vi "ET_Example.vi"() -> ()   [LabVIEW 2016]
uses:
  Source/Methods/Envelope Tracking/Typedefs/Detrough Configuration.ctl
  Source/Methods/Envelope Tracking/Typedefs/Detrough Type.ctl
  Source/SG/Typedefs/Instrument Configuration.ctl
  <instrlib>/niRFSG/niRFSG.llb/niRFSG Ref Clock Sources.ctl
  Source/Common/Local Oscillator Sharing Mode.ctl
  Source/Methods/Envelope Tracking/Typedefs/Synchronization Configuration.ctl
  Source/Methods/Envelope Tracking/Typedefs/Envelope Generator Configuration.ctl
  Source/Methods/Envelope Tracking/Typedefs/Tracker Configuration.ctl
  Source/Methods/Envelope Tracking/Typedefs/Lookup Table Configuration.ctl
  <instrlib>/niRFSG/niRFSG.llb/niRFSG Exported Signal Destinations.ctl
  Source/SG/SG.lvlib
  Source/Methods/Envelope Tracking/Envelope Tracking.lvlib
  Source/Common/Common.lvlib
panel:
  in  "stop":bool
  out "Status":string="Initializing..."
  out "error out":errorcluster {"code" format="%.0x"}
  in  "Configuration":T1(tab)
  in  "RF Signal Generator":refnum<k15>="5840"
  in  "Tracker Signal Generator":refnum<k15>="5820"
  in  "Waveform File Path":path=path "C:/Users/Public/Documents/National Instruments/RFIC Test Software/Waveforms/LTE_FDD_DL_1x20MHz_TM11_OS4.tdms"
  in  "Synchronization Configuration":T2={"RF Delay Range (s)"=1.9999999949504854e-06, "RF Delay (s)"=0.0} {"RF Delay (s)" format="%#_6p"; "RF Delay Range (s)" format="%#_6p"}
  in  "SG Configuration":T3={"SelectedPorts"="", "Reference Clock Source"="PXI_CLK", "Carrier Frequency (Hz)"=1000000000.0, "DUT Average Input Power (dBm)"=-10.0, "External Attenuation (dB)"=0.0, "LO Sharing Mode"=enum."Automatic"} {"Carrier Frequency (Hz)" format="%#_6p"}
  in  "Envelope Generator Configuration":T6={"Reference Clock Source"="PXI_CLK"}
  in  "Tracker Configuration":T7={"Input Impedance (Ohms)"=1000000.0, "Common Mode Offset (V)"=1.0, "Gain (V/V)"=2.5, "Output Offset (V)"=2.55} {"Input Impedance (Ohms)" format="%#_6p"}
  in  "Tracker Start Trigger Export":T8="PFI0"
  in  "Envelope Method":enum32{"Detrough", "LUT"}(tab)=enum."LUT"
  in  "Detrough Configuration":T9={"Type"=enum."Exponential", "Minimum Voltage (V)"=1.5, "Maximum Voltage (V)"=3.5, "Exponent"=1.2000000476837158}
  in  "Lookup Table Configuration":T11={"DUT Average Input Power (dBm)"=0.0, "DUT Input Power (dBm)"=array[1024 elements], "Supply Voltage (V)"=array[1024 elements]}
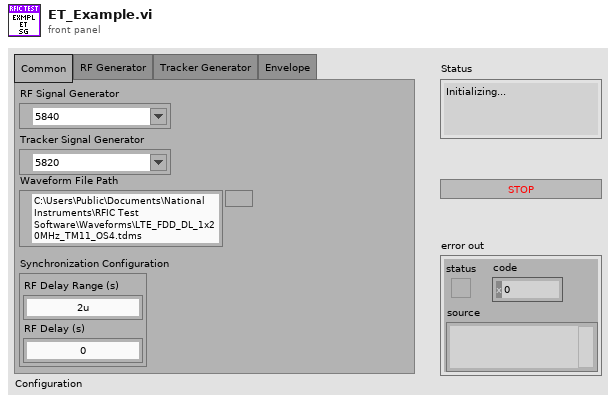
[diagram p1: front panel]
types:
  T1 = enum32{"Common", "RF Generator", "Tracker Generator", "Envelope"}
  T2 = typedef "Envelope Tracking.lvlib/Synchronization Configuration.ctl" = cluster{"RF Delay Range (s)":dbl, "RF Delay (s)":dbl}
  T3 = typedef "SG.lvlib/Instrument Configuration.ctl" = cluster{"SelectedPorts":string, "Reference Clock Source":T4, "Carrier Frequency (Hz)":dbl, "DUT Average Input Power (dBm)":dbl, "External Attenuation (dB)":dbl, "LO Sharing Mode":T5}
  T4 = typedef "niRFSG Ref Clock Sources.ctl" = string
  T5 = typedef "Common.lvlib/Local Oscillator Sharing Mode.ctl" = enum16{"Automatic", "None"}
  T6 = typedef "Envelope Tracking.lvlib/Envelope Generator Configuration.ctl" = cluster{"Reference Clock Source":T4}
  T7 = typedef "Envelope Tracking.lvlib/Tracker Configuration.ctl" = cluster{"Input Impedance (Ohms)":dbl, "Common Mode Offset (V)":dbl, "Gain (V/V)":dbl, "Output Offset (V)":dbl}
  T8 = typedef "niRFSG Exported Signal Destinations.ctl" = string
  T9 = typedef "Envelope Tracking.lvlib/Detrough Configuration.ctl" = cluster{"Type":T10, "Minimum Voltage (V)":dbl, "Maximum Voltage (V)":dbl, "Exponent":dbl}
  T10 = typedef "Envelope Tracking.lvlib/Detrough Type.ctl" = enum16{"Exponential", "Cosine", "Power"}
  T11 = typedef "Envelope Tracking.lvlib/Lookup Table Configuration.ctl" = cluster{"DUT Average Input Power (dBm)":dbl, "DUT Input Power (dBm)":sgl[], "Supply Voltage (V)":sgl[]}
  T12 = typedef "Common.lvlib/Waveform.ctl" = cluster{"Name":string, "Data":refnum<data-value>, "Signal Bandwidth (Hz)":dbl, "PAPR (dB)":dbl, "Burst Length (s)":dbl, "Sample Rate":dbl, "Burst Start Locations":i32[], "Burst Stop Locations":i32[], "Idle Duration Present?":bool, "Runtime Scaling":dbl, "Script":string}
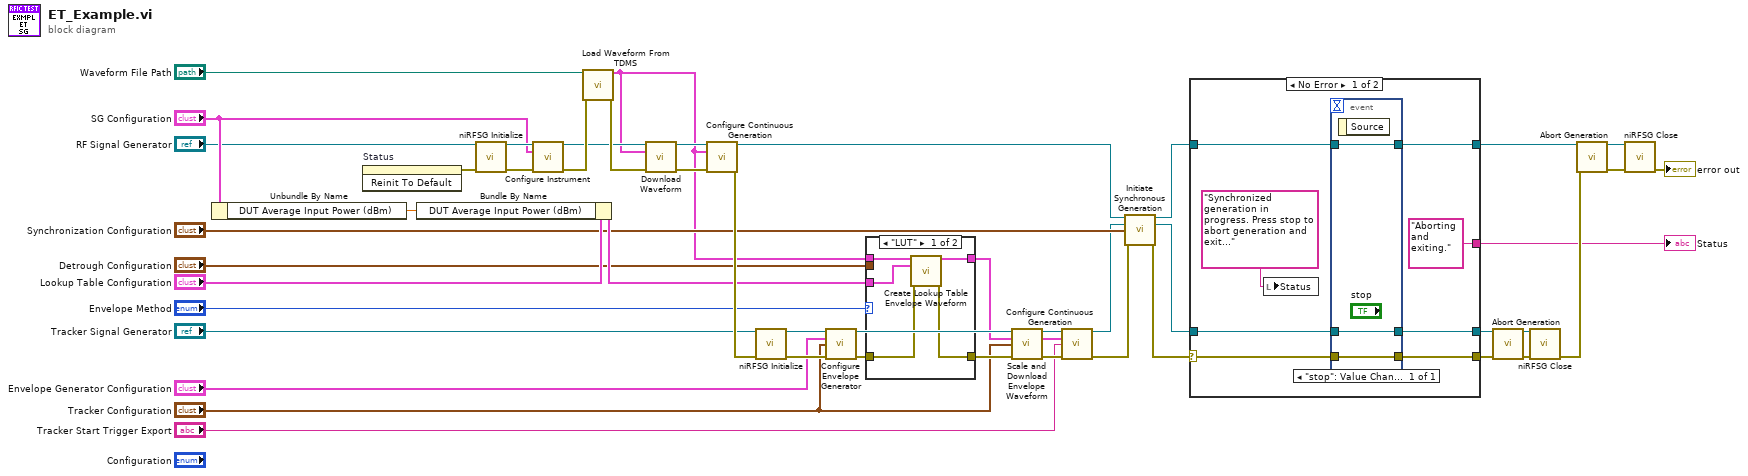
[diagram p0: block diagram]
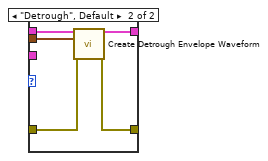
[diagram p2: hidden frame]
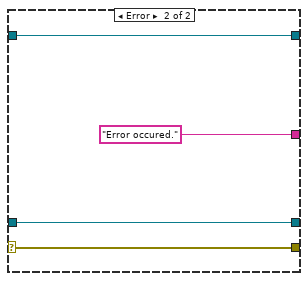
[diagram p3: hidden frame]
diagram:
  n1 = Unbundle By Name("SG Configuration") -> ("DUT Average Input Power (dBm)"=w3:dbl)
  n2 = invoke on="Status" class="Str" method="Reinit To Default"() -> (error out=w32:errorcluster)  [unwired: 3 in, 2 out]
  n3 = Bundle By Name(cluster="Lookup Table Configuration", "DUT Average Input Power (dBm)"=w3) -> (w30:T11)
  n4 = call <instrlib>:"niRFSG Initialize.vi"("resource name"="RF Signal Generator", "error in"=w32) -> ("instrument handle"=w27:refnum<k15>, "error out"=w48:errorcluster)  [unwired: 12 in]
  n5 = call "Configure Instrument.vi"("RFSG Session In"=w27, "SG Configuration"="SG Configuration", "error in (no error)"=w48) -> ("RFSG Session Out"=w26:refnum<k15>, "error out"=w40:errorcluster)  [unwired: 11 in]
  n6 = call "Load Waveform From TDMS.vi"("TDMS File Path"="Waveform File Path", "error in (no error)"=w40) -> ("Waveform"=w1:T12, "error out"=w39:errorcluster)  [unwired: 12 in]
  n7 = call "Download Waveform.vi"("RFSG handle"=w26, "Waveform In"=w1, "error in (no error)"=w39) -> ("RFSG handle out"=w25:refnum<k15>, "error out"=w47:errorcluster)  [unwired: 11 in]
  n8 = call "Configure Continuous Generation.vi"("RFSG handle"=w25, "Waveform in"=w1, "error in"=w47) -> ("RFSG handle out"=w18:refnum<k15>, "error out"=w38:errorcluster)  [unwired: 10 in, 1 out]
  n9 = call <instrlib>:"niRFSG Initialize.vi"("resource name"="Tracker Signal Generator", "error in"=w38) -> ("instrument handle"=w24:refnum<k15>, "error out"=w46:errorcluster)  [unwired: 12 in]
  n10 = call "Configure Envelope Generator.vi"("Envelope Generator Handle in"=w24, "Envelope Generator Configuration"="Envelope Generator Configuration", "Tracker Configuration"="Tracker Configuration", "error in"=w46) -> ("Envelope Generator Handle out"=w23:refnum<k15>, "error out"=w44:errorcluster)  [unwired: 10 in]
  n11 = case shown="\"LUT\"" "Envelope Method" {
    tunnel: w44 -> [w53 w58]
    tunnel: [w52 w57] -> w43
    tunnel: [w51 w56] -> w21
    tunnel: w1 -> [w50 w55]
    tunnel: "Detrough Configuration" -> [_ w54]
    tunnel: w30 -> [w49 _]
    frame "LUT" {
      n12 = call "Create Lookup Table Envelope Waveform.vi"("Reference Waveform"=w50, "Lookup Table Configuration"=w49, "error in (no error)"=w53) -> ("Lookup Table Envelope Waveform"=w51:T12, "error out"=w52:errorcluster)  [unwired: 11 in]
    }
    frame "Detrough", Default {
      n13 = call "Create Detrough Envelope Waveform.vi"("Reference Waveform"=w55, "Detrough Configuration"=w54, "error in (no error)"=w58) -> ("Detrough Envelope Waveform"=w56:T12, "error out"=w57:errorcluster)  [unwired: 11 in]
    }
  }
  n14 = call "Scale and Download Envelope Waveform.vi"("Envelope Generator Handle in"=w23, "Envelope Waveform"=w21, "Tracker Configuration"="Tracker Configuration", "error in (no error)"=w43) -> ("Envelope Generator Handle out"=w22:refnum<k15>, "Scaled Envelope Waveform"=w20:T12, "error out"=w45:errorcluster)  [unwired: 9 in]
  n15 = call "Configure Continuous Generation.vi"("RFSG handle"=w22, "Waveform in"=w20, "Waveform Start Trigger Export"="Tracker Start Trigger Export", "error in"=w45) -> ("RFSG handle out"=w14:refnum<k15>, "error out"=w37:errorcluster)  [unwired: 9 in, 1 out]
  n16 = call "Initiate Synchronous Generation.vi"("RF Generator Handle in"=w18, "Envelope Generator Handle in"=w14, "Synchronization Configuration"="Synchronization Configuration", "error in (no error)"=w37) -> ("RF Generator Handle out"=w7:refnum<k15>, "Envelope Generator Handle out"=w9:refnum<k15>, "error out"=w35:errorcluster)  [unwired: 9 in]
  n17 = case shown="No Error" w35 {
    selector: w35 -> [w66 w73]
    tunnel: [w63 w72] -> w10
    tunnel: w9 -> [w64 w72]
    tunnel: [w65 w73] -> w34
    tunnel: [w62 w71] -> w8
    tunnel: w7 -> [w61 w71]
    tunnel: ["Aborting and exiting." ("Status") "Error occured." ("Status")] -> w5
    frame No Error {
      n18 = local write "Status"("Synchronized generation in progress. Press stop to abort generation and exit...") -> ()
      n19 = event shown="[0] \"stop\": Value Change" {
        selector: _ -> [_]
        dyn-events: _ -> [_]
        timeout: _ -> [_]
        tunnel: [w68] -> w63
        tunnel: w64 -> [w68]
        tunnel: [w69] -> w65
        tunnel: w66 -> [w69]
        tunnel: w61 -> [w67]
        tunnel: [w67] -> w62
        event "stop": Value Change {
          n20 = event-data() -> ()  [unwired: 1 in, 1 out]
        }
      }
    }
    frame Error {
    }
  }
  "Status" <- w5
  n21 = call "Abort Generation.vi"("RFSG handle"=w10, "error in (no error)"=w34) -> ("RFSG handle out"=w15:refnum<k15>, "error out"=w41:errorcluster)  [unwired: 12 in]
  n22 = call <instrlib>:"niRFSG Close.vi"("instrument handle"=w15, "error in"=w41) -> ("error out"=w36:errorcluster)  [unwired: 13 in]
  n23 = call "Abort Generation.vi"("RFSG handle"=w8, "error in (no error)"=w36) -> ("RFSG handle out"=w16:refnum<k15>, "error out"=w42:errorcluster)  [unwired: 12 in]
  n24 = call <instrlib>:"niRFSG Close.vi"("instrument handle"=w16, "error in"=w42) -> ("error out"=→"error out":errorcluster)  [unwired: 13 in]
